vi "Create NI 9227.vi"(8 "error in":errorcluster, 11 "channel settings":T1[](array[typedef])) -> (0 "error out":errorcluster, 3 "NI 9227 out":refnum<class "NI 9227.lvclass">)   [LabVIEW 2020, in "Scan Engine Scripting.lvlib" / "NI 9227.lvclass"]
doc: "Creates and configures an instance of a NI-9227 analog input module that can be used to set a slot in a Scan Engine custom device chassis."
uses:
  NI 9227.lvclass
  Mode Classes/Controls/analog channel settings.ctl
  Mode Classes/Analog Input Arms Mode/Analog Input Arms Mode.lvclass
  C:/jenkins/workspace/ercat-custom-device_release_20.4/Custom Device Source/Scripting/Modules/Mode Classes/Mode/Mode.lvclass
  4ab162af-d640-44eb-9977-177cf6a3db57.vi
  Scan Engine Scripting.lvlib
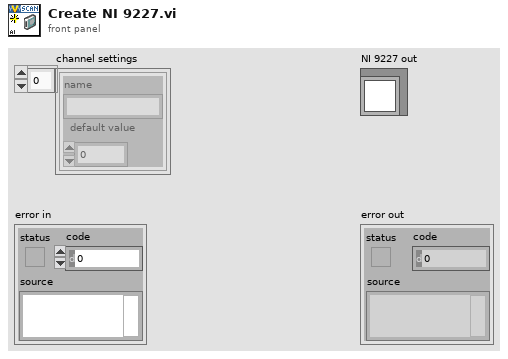
[diagram p1: front panel]
types:
  T1 = typedef "Scan Engine Scripting.lvlib/analog channel settings.ctl" = cluster{"name":string, "default value":dbl}
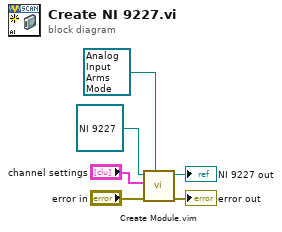
[diagram p0: block diagram]
diagram:
  n1 = call "Create Module.vim"("mode"=refnum<class "Analog Input Arms Mode.lvclass"> refnum ("Scan Engine Scripting.lvlib:Analog Input Arms Mode.lvclass"), "error in"="error in", "channel settings"="channel settings", "module in"=refnum<class "NI 9227.lvclass"> refnum ("Scan Engine Scripting.lvlib:NI 9225.lvclass")) -> ("error out"=→"error out":errorcluster, "module out"=→"NI 9227 out":refnum<class "NI 9227.lvclass">)  [unwired: 6 in]
